vi "Fetch GPM Repo.vi"(8 "error in (no error)":errorcluster) -> (0 "error out":errorcluster, 3 "Repo":refnum<class "Repo.lvclass">)   [LabVIEW 2020, in "Packages.lvlib" / "GPM.lvlib"]
uses:
  GPM.lvlib
  Repo_class/Repo.lvclass
  Repo_class/Repo.lvclass/Repo.ctl
  G Package_class/G Package.lvclass
  C:/git/GCentral/Website/LV WebServices/Libraries/Packages/Package_class/Package.lvclass
  Package Version_class/Package Version.lvclass/Package Version.ctl
  Package_class/Package.lvclass/Package.ctl
  Package Version_class/Read DisplayName.vi
  Package_class/Write Name.vi
  Package_class/Write RepoName.vi
  Package_class/Write RepoType.vi
  Package_class/Write DisplayName.vi
  Package_class/Write Versions.vi
  Repo_class/Read Name.vi
  Repo_class/Read RepoType.vi
  Repo_class/Write Packages.vi
  <vilib>/httpClient/LabVIEWHTTPClient.lvlib
  Package Version_class/Package Version.lvclass
  WSsupport/WSsupport.lvlib
panel:
  out "Progress":u8(slide) scale=0.0..100.0
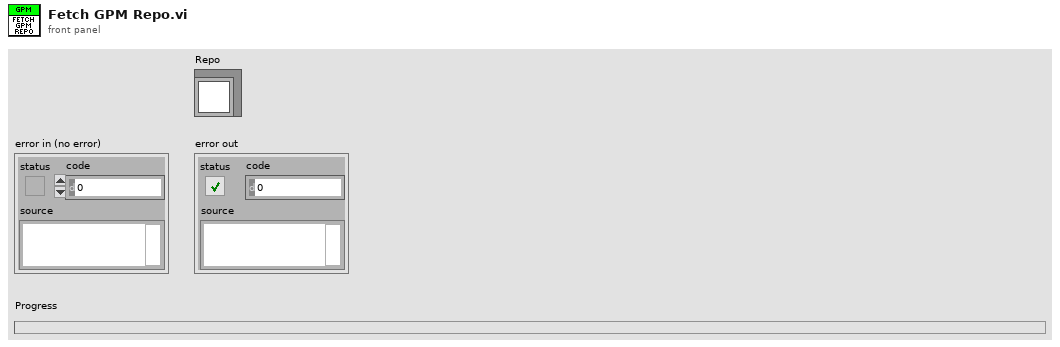
[diagram p1: front panel]
types:
  T1 = typedef "Packages.lvlib/Repo.lvclass/RepoType--enum.ctl" = enum16{"VIPM", "NIPM", "GPM"}
  T2 = typedef "Packages.lvlib/Package--cluster.ctl" = cluster{"Name":string, "Versions":string[]}
  T3 = typedef "LabVIEWHTTPClient.lvlib/ClientHandle.ctl" = refnum<k1>
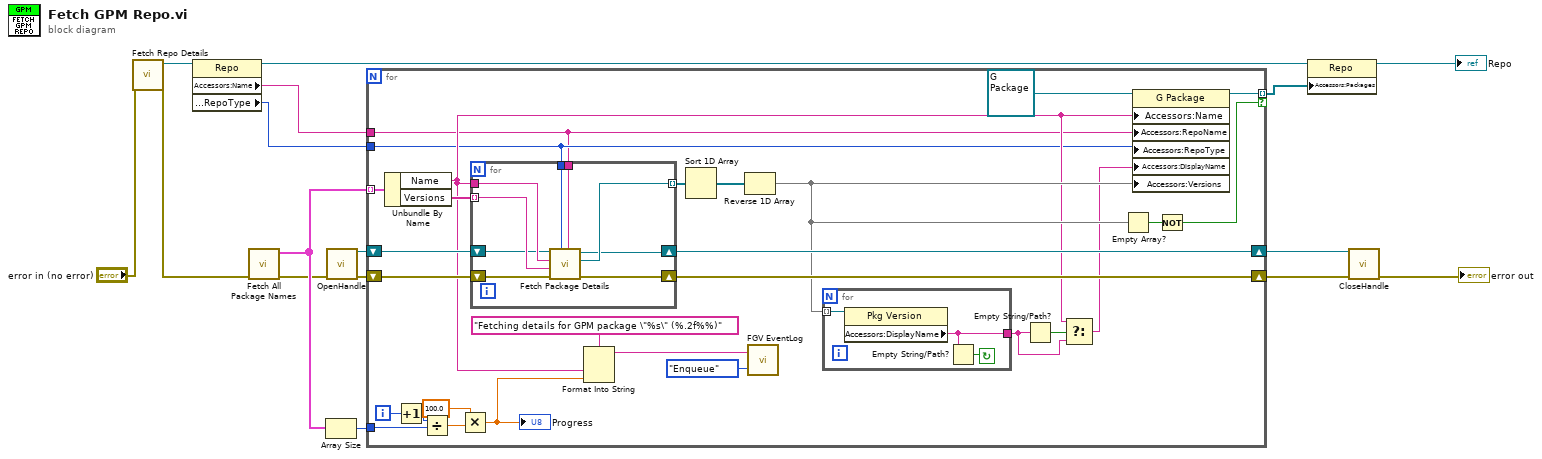
[diagram p0: block diagram]
diagram:
  n1 = call "Fetch Repo Details.vi"("error in (no error)"="error in (no error)") -> ("error out"=w7:errorcluster, "Repo"=w10:refnum<class "Repo.lvclass">)  [unwired: 9 in]
  n2 = property class="Repo"(reference=w10) -> (reference out=w12:refnum<class "Repo.lvclass">, "Accessors:Name"=w11:string, "Accessors:RepoType"=w5:T1)  [unwired: 1 in, 1 out]
  n3 = call "Fetch All Package Names.vi"("error in (no error)"=w7) -> ("error out"=w6:errorcluster, "All Packages"=w8:T2[])  [unwired: 9 in]
  n4 = Array Size(array=w8) -> (size(s)=w13:i32)
  n5 = call <vilib>:"OpenHandle.vi"("error in (no error)"=w6) -> ("client handle out"=w3:T3, "error out"=w4:errorcluster)  [unwired: 13 in]
  n6 = for {
    shift-right: [w28] -> w16
    shift-left: w4 -> [w29]
    tunnel: w8 -> [w44] mode=indexing
    tunnel: [w41] -> w14 mode=indexing if=w33
    tunnel: w13 -> [w39]
    tunnel: w5 -> [w18]
    tunnel: w11 -> [w17]
    shift-right: [w30] -> w1
    shift-left: w3 -> [w31]
    i -> [w40]
    n7 = Unbundle By Name(w44) -> ("Name"=w20:string, "Versions"=w43:string[])
    n8 = Increment(x=w40) -> (x+1=w38:i32)
    n9 = Divide(x=w38, y=w39) -> (x/y=w37:dbl)
    n10 = Multiply(x=100.0, y=w37) -> (x*y=w19:dbl)
    "Progress" <- w19
    n11 = for {
      tunnel: w20 -> [w53]
      tunnel: w43 -> [w55] mode=indexing
      tunnel: [w54] -> w35 mode=indexing
      shift-right: [w51] -> w30
      shift-left: w31 -> [w52]
      shift-right: [w50] -> w28
      shift-left: w29 -> [w56]
      tunnel: w18 -> [w49]
      tunnel: w17 -> [w48]
      n12 = call "Fetch Package Details.vi"("RepoName"=w48, "RepoType"=w49, "error in (no error)"=w56, "Package Version"=w55, "Package Name"=w53, "HTTP handle in"=w52) -> ("error out"=w50:errorcluster, "Pkg Version"=w54:refnum<class "Package Version.lvclass">, "HTTP handle out"=w51:T3)  [unwired: 3 in]
    }
    n13 = Format Into String(format string="Fetching details for GPM package \"%s\" (%.2f%%)", w20, w19) -> (resulting string=w22:string)  [unwired: 2 in, 1 out]
    n14 = Sort 1D Array(array=w35) -> (sorted array=w32:refnum<class "Package Version.lvclass">[])
    n15 = Reverse 1D Array(array=w32) -> (reversed array=w27:refnum<class "Package Version.lvclass">[])
    n16 = call "FGV EventLog.vi"("Action"=enum16{"Reset", "Enqueue", "Dequeue"}."Enqueue", "String to log"=w22) -> ()  [unwired: 1 in, 1 out]
    n17 = for {
      tunnel: [w46] -> w25
      tunnel: w27 -> [w47] mode=indexing
      stop <- w45 continue-if-true
      n18 = property class="Pkg Version"(reference=w47) -> ("Accessors:DisplayName"=w46:string)  [unwired: 1 in, 2 out]
      n19 = Empty String/Path?(string/path=w46) -> (empty?=w45:bool)
    }
    n20 = Empty String/Path?(string/path=w25) -> (empty?=w26:bool)
    n21 = Select(t=w20, s=w26, f=w25) -> (s? t:f=w24:string)
    n22 = Empty Array?(array=w27) -> (empty?=w34:bool)
    n23 = property class="G Package"(reference=refnum<class "G Package.lvclass"> refnum ("Packages.lvlib:G Package"), "Accessors:Name"=w20, "Accessors:RepoName"=w17, "Accessors:RepoType"=w18, "Accessors:DisplayName"=w24, "Accessors:Versions"=w27) -> (reference out=w41:refnum<class "G Package.lvclass">)  [unwired: 1 in, 1 out]
    n24 = Not(x=w34) -> (.not. x?=w33:bool)
  }
  n25 = property class="Repo"(reference=w12, "Accessors:Packages"=w14) -> (reference out=→"Repo":refnum<class "Repo.lvclass">)  [unwired: 1 in, 1 out]
  n26 = call <vilib>:"CloseHandle.vi"("client handle"=w1, "error in (no error)"=w16) -> ("error out"=→"error out":errorcluster)  [unwired: 13 in]
